vi "Update Joints.vi"(8 "error in (no error)":errorcluster, 9 "Joints":sgl[](array[numeric]), 10 "Joint Array":T1[](array[typedef])) -> (0 "error out":errorcluster)   [LabVIEW 2015]
doc: "The VI updates the joints of the robot."
uses:
  <vilib>/robotics/Kinematics/Plotting/Joint Control.ctl
  <vilib>/robotics/Kinematics/Plotting/Joint Type.ctl
  <vilib>/Utility/AngleManip/Degrees to Radians (Scalar DBL).vi
  <vilib>/picture/3D Picture Control/NI_3D Picture Control.lvlib
  <vilib>/Utility/AngleManip/NI_AngleManipulation.lvlib
  <vilib>/robotics/Kinematics/Plotting/NI_Robotics_3DKinematics.lvlib
panel:
  in  "Scale (1)":dbl=1.0
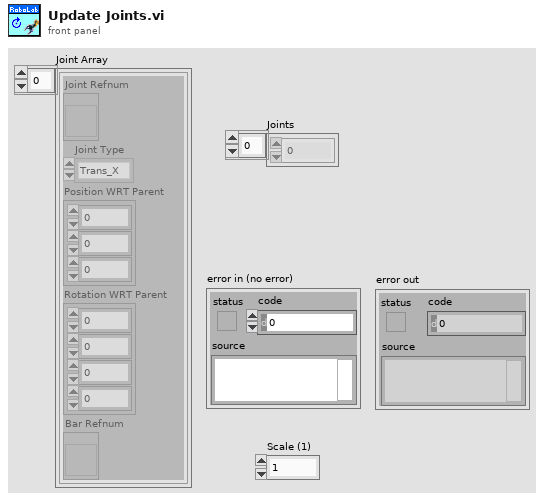
[diagram p1: front panel]
types:
  T1 = typedef "NI_Robotics_3DKinematics.lvlib/Joint Control.ctl" = cluster{"Joint Refnum":refnum<vi>, "Joint Type":T2, "Position WRT Parent":dbl[], "Rotation WRT Parent":dbl[], "Bar Refnum":refnum<vi>}
  T2 = typedef "NI_Robotics_3DKinematics.lvlib/Joint Type.ctl" = enum16{"Trans_X", "Trans_Y", "Trans_Z", "Rot_X", "Rot_Y", "Rot_Z", "None"}
  T3 = cluster{"Rotation WRT Parent[0]":dbl, "Rotation WRT Parent[1]":dbl, "Rotation WRT Parent[2]":dbl}
  T4 = cluster{"Numeric":dbl, "Numeric":dbl, "Numeric":dbl}
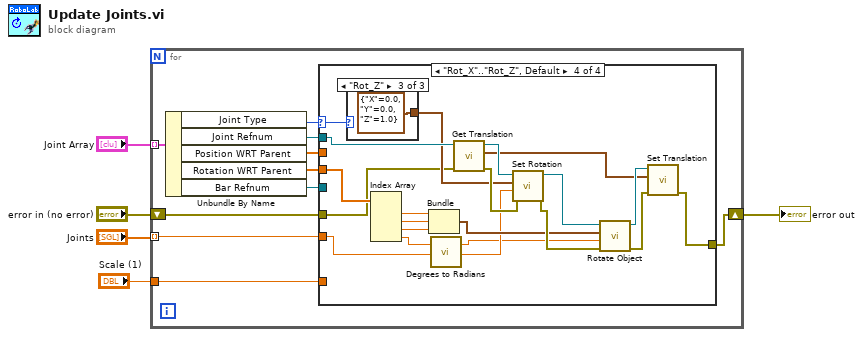
[diagram p0: block diagram]
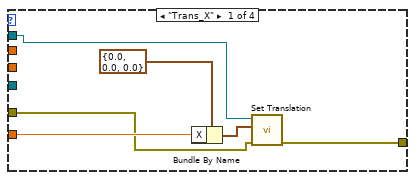
[diagram p2: hidden frame]
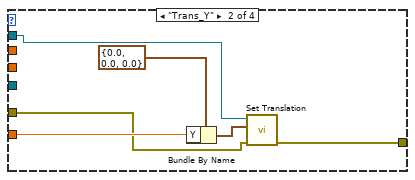
[diagram p3: hidden frame]
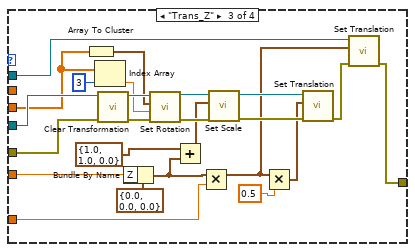
[diagram p4: hidden frame]
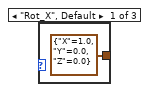
[diagram p5: hidden frame]
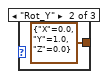
[diagram p6: hidden frame]
diagram:
  n1 = for {
    tunnel: "Joint Array" -> [w14] mode=indexing
    tunnel: "Joints" -> [w15] mode=indexing
    shift-right: [w11] -> w2
    shift-left: "error in (no error)" -> [w8]
    tunnel: "Scale (1)" -> [w6]
    n2 = Unbundle By Name(w14) -> ("Joint Type"=w9:T2, "Joint Refnum"=w10:refnum<vi>, "Position WRT Parent"=w12:dbl[], "Rotation WRT Parent"=w13:dbl[], "Bar Refnum"=w7:refnum<vi>)
    n3 = case shown="\"Rot_X\"..\"Rot_Z\", Default" w9 {
      selector: w9 -> [_ _ _ w58]
      tunnel: w15 -> [w19 w27 w50 w54]
      tunnel: [w20 w25 w40 w63] -> w11
      tunnel: w13 -> [_ _ w32 w71]
      tunnel: w12 -> [_ _ _ _]
      tunnel: w10 -> [w17 w23 w42 w59]
      tunnel: w8 -> [w16 w22 w35 w55]
      tunnel: w7 -> [_ _ w36 _]
      tunnel: w6 -> [_ _ w28 _]
      frame "Trans_X" {
        n4 = Bundle By Name(cluster=cluster{"X":sgl, "Y":sgl, "Z":sgl} {"X"=0.0, "Y"=0.0, "Z"=0.0} ("Translation"), "X"=w19) -> (w21:cluster{"X":sgl, "Y":sgl, "Z":sgl})
        n5 = call <vilib>:"Set Translation.vi"("error in (no error)"=w16, "Translation"=w21, "Scene Object"=w17) -> ("error out"=w20:errorcluster)  [unwired: 8 out]
      }
      frame "Trans_Y" {
        n6 = Bundle By Name(cluster=cluster{"X":sgl, "Y":sgl, "Z":sgl} {"X"=0.0, "Y"=0.0, "Z"=0.0} ("Translation"), "Y"=w27) -> (w26:cluster{"X":sgl, "Y":sgl, "Z":sgl})
        n7 = call <vilib>:"Set Translation.vi"("error in (no error)"=w22, "Translation"=w26, "Scene Object"=w23) -> ("error out"=w25:errorcluster)  [unwired: 8 out]
      }
      frame "Trans_Z" {
        n8 = Array To Cluster(array=w32) -> (cluster=w34:T3)
        n9 = Index Array(array=w32, index=3) -> (element=w31:dbl)
        n10 = call <vilib>:"Clear Transformation.vi"("error in (no error)"=w35, "Object Refnum In"=w36) -> ("error out"=w49:errorcluster, "Object Refnum Out"=w48:refnum<vi>)  [unwired: 8 in]
        n11 = Bundle By Name(cluster=cluster{"X":sgl, "Y":sgl, "Z":sgl} {"X"=0.0, "Y"=0.0, "Z"=0.0} ("Translation"), "Z"=w50) -> (w39:cluster{"X":sgl, "Y":sgl, "Z":sgl})
        n12 = call <vilib>:"Set Rotation.vi"("error in (no error)"=w49, "Angle"=w31, "Axis"=w34, "Scene Object"=w48) -> ("error out"=w46:errorcluster, "Rotated Scene Object"=w47:refnum<vi>)  [unwired: 6 in]
        n13 = Add(x=cluster{"X":sgl, "Y":sgl, "Z":sgl} {"X"=1.0, "Y"=1.0, "Z"=0.0} ("Translation"), y=w39) -> (x+y=w38:cluster{"X":sgl, "Y":sgl, "Z":sgl})
        n14 = Multiply(x=w39, y=w28) -> (x*y=w29:cluster{"X":dbl, "Y":dbl, "Z":dbl})
        n15 = call <vilib>:"Set Scale.vi"("error in (no error)"=w46, "Scale"=w38, "Scene Object"=w47) -> ("error out"=w44:errorcluster, "Scaled Object"=w45:refnum<vi>)  [unwired: 7 in]
        n16 = Multiply(x=w29, y=0.5) -> (x*y=w43:cluster{"X":dbl, "Y":dbl, "Z":dbl})
        n17 = call <vilib>:"Set Translation.vi"("error in (no error)"=w44, "Translation"=w43, "Scene Object"=w45) -> ("error out"=w41:errorcluster)  [unwired: 7 in, 1 out]
        n18 = call <vilib>:"Set Translation.vi"("error in (no error)"=w41, "Translation"=w29, "Scene Object"=w42) -> ("error out"=w40:errorcluster)  [unwired: 8 out]
      }
      frame "Rot_X".."Rot_Z", Default {
        n19 = case shown="\"Rot_Z\"" w58 {
          tunnel: [cluster{"X":sgl, "Y":sgl, "Z":sgl} {"X"=1.0, "Y"=0.0, "Z"=0.0} ("Axis") cluster{"X":sgl, "Y":sgl, "Z":sgl} {"X"=0.0, "Y"=1.0, "Z"=0.0} ("Axis") cluster{"X":sgl, "Y":sgl, "Z":sgl} {"X"=0.0, "Y"=0.0, "Z"=1.0} ("Axis")] -> w57
          frame "Rot_X", Default {
          }
          frame "Rot_Y" {
          }
          frame "Rot_Z" {
          }
        }
        n20 = Index Array(array=w71) -> (element #1=w68:dbl, element #2=w67:dbl, element #3=w66:dbl, element #4=w52:dbl)  [unwired: 4 in]
        n21 = Bundle("Numeric"=w68, "Numeric"=w67, "Numeric"=w66) -> (w56:T4)  [unwired: 1 in]
        n22 = call-poly <vilib>:"Degrees to Radians.vi"("angle (deg)"=w52) -> ("angle (rad)"=w53:dbl)  [unwired: 2 in]
        n23 = call <vilib>:"Get Translation.vi"("error in (no error)"=w55, "Scene Object"=w59) -> ("error out"=w64:errorcluster, "Transformation:Get Translation"=w60:cluster{"X":sgl, "Y":sgl, "Z":sgl}, "Scene Object"=w65:refnum<vi>)  [unwired: 7 in]
        n24 = call <vilib>:"Set Rotation.vi"("error in (no error)"=w64, "Angle"=w54, "Axis"=w57, "Scene Object"=w65) -> ("error out"=w70:errorcluster, "Rotated Scene Object"=w69:refnum<vi>)  [unwired: 6 out]
        n25 = call <vilib>:"Rotate Object.vi"("error in (no error)"=w70, "Angle"=w53, "Axis"=w56, "Scene.Object In"=w69) -> ("error out"=w62:errorcluster, "Scene.Object Out"=w61:refnum<vi>)  [unwired: 6 in]
        n26 = call <vilib>:"Set Translation.vi"("error in (no error)"=w62, "Translation"=w60, "Scene Object"=w61) -> ("error out"=w63:errorcluster)  [unwired: 7 in, 1 out]
      }
    }
  }
  "error out" <- w2
